vi "Heating second step (SILAR).vi"(0 "Arduino Resource In":T1={"VISA resource"="", "Board Type"=enum."Uno", "Connection Type"=enum."USB / Serial", "Bytes Per Packet (15)"=15}, 2 "Turn on_off":bool, 3 "Время всего процесса":dbl, 5 "Error In":errorcluster, 6 "Необходимая температура":dbl[](array[numeric])=[1.0, 1.0, 1.0, 1.0], 8 "Текущая температура":dbl[](array[numeric])=[1.0, 1.0, 1.0, 1.0]) -> ()   [LabVIEW 2012]
uses:
  <vilib>/LabVIEW Interface for Arduino/Type Defs/Arduino Resource.ctl
  <vilib>/LabVIEW Interface for Arduino/Type Defs/Board Type.ctl
  <vilib>/LabVIEW Interface for Arduino/LabVIEW Interface for Arduino.lvlib
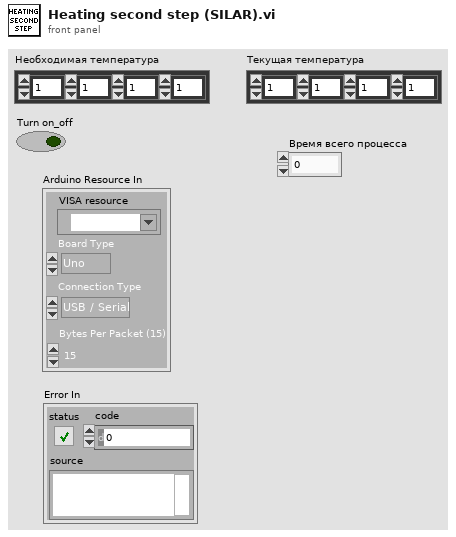
[diagram p1: front panel]
types:
  T1 = typedef "LabVIEW Interface for Arduino.lvlib/Arduino Resource.ctl" = cluster{"VISA resource":refnum<visa-resource-name>, "Board Type":T2, "Connection Type":enum8{"USB / Serial"}, "Bytes Per Packet (15)":u8}
  T2 = typedef "LabVIEW Interface for Arduino.lvlib/Board Type.ctl" = enum16{"Uno", "Dimuelanove w/Atmega 328", "Mega 2560"}
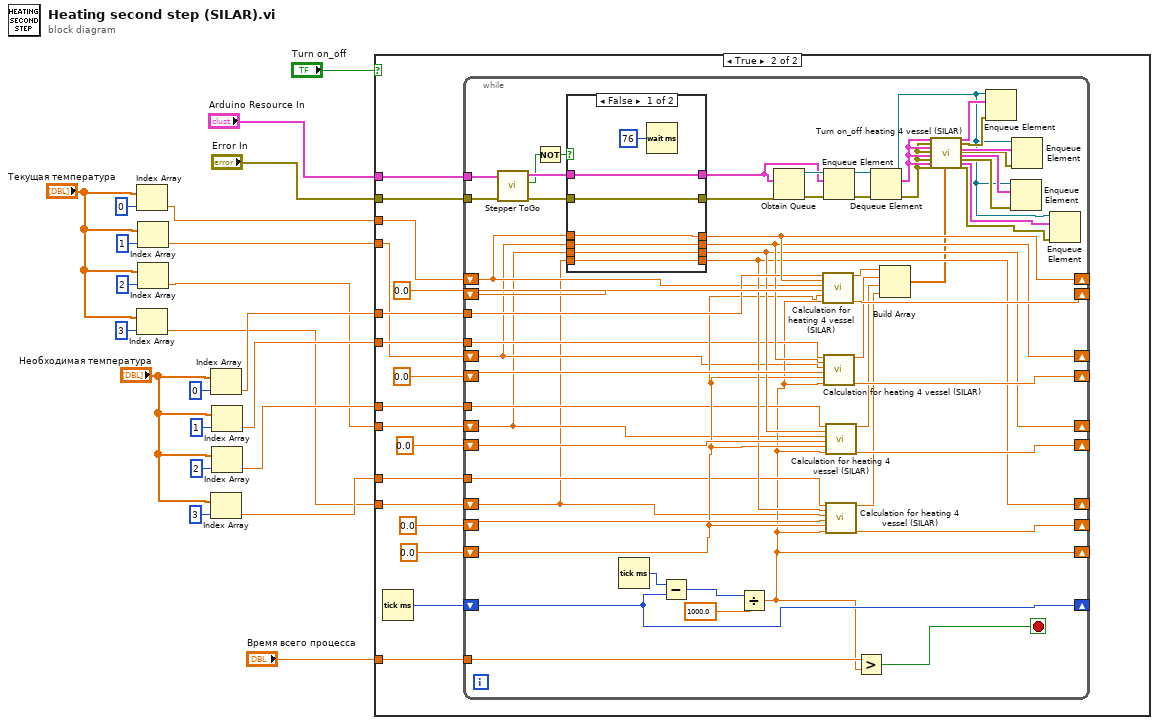
[diagram p0: block diagram]
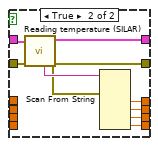
[diagram p3: hidden frame]
diagram:
  n1 = Index Array(array="Текущая температура", index=0) -> (element=w5:dbl)
  n2 = Index Array(array="Текущая температура", index=3) -> (element=w2:dbl)
  n3 = Index Array(array="Текущая температура", index=1) -> (element=w4:dbl)
  n4 = Index Array(array="Текущая температура", index=2) -> (element=w3:dbl)
  n5 = Index Array(array="Необходимая температура", index=0) -> (element=w17:dbl)
  n6 = Index Array(array="Необходимая температура", index=3) -> (element=w14:dbl)
  n7 = Index Array(array="Необходимая температура", index=1) -> (element=w16:dbl)
  n8 = Index Array(array="Необходимая температура", index=2) -> (element=w15:dbl)
  n9 = case shown="True" "Turn on_off" {
    tunnel: "Arduino Resource In" -> [_ w39]
    tunnel: "Error In" -> [_ w38]
    tunnel: w17 -> [_ w36]
    tunnel: w16 -> [_ w30]
    tunnel: w15 -> [_ w29]
    tunnel: w14 -> [_ w28]
    tunnel: w5 -> [_ w27]
    tunnel: w4 -> [_ w26]
    tunnel: w3 -> [_ w25]
    tunnel: w2 -> [_ w24]
    tunnel: "Время всего процесса" -> [_ w23]
    frame False {
    }
    frame True {
      n10 = Tick Count (ms)() -> (millisecond timer value=w35:u32)
      n11 = while {
        tunnel: w39 -> [w55]
        tunnel: w38 -> [w56]
        shift-right: [w81] -> _
        shift-left: w27 -> [w47]
        shift-right: [w83] -> _
        shift-left: 0.0 ("Ts - суммарная температура") -> [w82]
        tunnel: w36 -> [w80]
        shift-right: [w73] -> _
        shift-left: w26 -> [w46]
        shift-right: [w77] -> _
        shift-left: 0.0 -> [w76]
        shift-right: [w72] -> _
        shift-left: w25 -> [w45]
        shift-right: [w78] -> _
        shift-left: 0.0 -> [w75]
        shift-right: [w71] -> _
        shift-left: w24 -> [w44]
        shift-right: [w79] -> _
        shift-left: 0.0 -> [w74]
        shift-right: [w67] -> _
        shift-left: w35 -> [w67]
        shift-right: [w49] -> _
        shift-left: 0.0 -> [w66]
        tunnel: w30 -> [w65]
        tunnel: w29 -> [w64]
        tunnel: w28 -> [w63]
        tunnel: w23 -> [w50]
        stop <- w48 stop-if-true
        n12 = call <vilib>:"Stepper ToGo.vi"("error in"=w56, "Arduino Resource"=w55) -> ("error out"=w53:errorcluster, "Steps Remaining?"=w51:bool, "Arduino Resource Out"=w54:T1)  [unwired: 6 in, 1 out]
        n13 = Not(x=w51) -> (.not. x?=w52:bool)
        n14 = case shown="False" w52 {
          tunnel: [w101 w111] -> w94
          tunnel: [w99 w110] -> w81
          tunnel: [w98 w109] -> w73
          tunnel: [w97 w108] -> w72
          tunnel: [w96 w107] -> w71
          tunnel: [w100 w105] -> w57
          tunnel: w54 -> [w101 w104]
          tunnel: w53 -> [w100 w103]
          tunnel: w47 -> [w99 _]
          tunnel: w46 -> [w98 _]
          tunnel: w45 -> [w97 _]
          tunnel: w44 -> [w96 _]
          frame False {
            n15 = Wait (ms)(milliseconds to wait=u32 76) -> ()  [unwired: 1 out]
          }
          frame True {
            n16 = call "Reading temperature (SILAR).vi"("error in"=w103, "Arduino Resource in"=w104) -> ("error out"=w105:errorcluster, "Arduino Resource"=w111:T1, "read buffer"=w106:string)  [unwired: 7 in]
            n17 = Scan From String(input string=w106, error in=w105) -> (output 1=w110:dbl, output 2=w109:dbl, output 3=w108:dbl, output 4=w107:dbl)  [unwired: 6 in, 3 out]
          }
        }
        n18 = Tick Count (ms)() -> (millisecond timer value=w70:u32)
        n19 = Subtract(x=w70, y=w67) -> (x-y=w68:u32)
        n20 = Divide(x=w68, y=1000.0) -> (x/y=w49:dbl)
        n21 = Obtain Queue(element data type=w94, error in (no error)=w57) -> (queue out=w95:refnum<queue>, error out=w40:errorcluster)  [unwired: 3 in, 1 out]
        n22 = call "Calculation for heating 4 vessel (SILAR).vi"("Tz - заданная температура"=w80, "Tt - текущая температура"=w81, "Ttp - текущая (прошлая) температура"=w47, "Tsp - суммарная (прошлая) температура"=w82, "tp - время прошлое"=w66, "tn - время настоящее"=w49) -> ("t1 - время во включенном состоянии"=w62:dbl, "Ts - суммарная температура"=w83:dbl)  [unwired: 12 in]
        n23 = Enqueue Element(queue=w95, element=w94, error in (no error)=w40) -> (queue out=w93:refnum<queue>, error out=w92:errorcluster)  [unwired: 1 in, 1 out]
        n24 = call "Calculation for heating 4 vessel (SILAR).vi"("Tz - заданная температура"=w65, "Tt - текущая температура"=w73, "Ttp - текущая (прошлая) температура"=w46, "Tsp - суммарная (прошлая) температура"=w76, "tp - время прошлое"=w66, "tn - время настоящее"=w49) -> ("t1 - время во включенном состоянии"=w60:dbl, "Ts - суммарная температура"=w77:dbl)  [unwired: 12 in]
        n25 = call "Calculation for heating 4 vessel (SILAR).vi"("Tz - заданная температура"=w64, "Tt - текущая температура"=w72, "Ttp - текущая (прошлая) температура"=w45, "Tsp - суммарная (прошлая) температура"=w75, "tp - время прошлое"=w66, "tn - время настоящее"=w49) -> ("t1 - время во включенном состоянии"=w59:dbl, "Ts - суммарная температура"=w78:dbl)  [unwired: 12 in]
        n26 = call "Calculation for heating 4 vessel (SILAR).vi"("Tz - заданная температура"=w63, "Tt - текущая температура"=w71, "Ttp - текущая (прошлая) температура"=w44, "Tsp - суммарная (прошлая) температура"=w74, "tp - время прошлое"=w66, "tn - время настоящее"=w49) -> ("t1 - время во включенном состоянии"=w58:dbl, "Ts - суммарная температура"=w79:dbl)  [unwired: 12 in]
        n27 = Greater?(x=w50, y=w49) -> (0:w48:bool)
        n28 = Dequeue Element(queue=w93, error in (no error)=w92) -> (queue out=w41:refnum<queue>, element=w91:T1, error out=w90:errorcluster)  [unwired: 1 in, 1 out]
        n29 = Build Array(w62, w60, w59, w58) -> (w61:dbl[])
        n30 = call "Turn on_off heating 4 vessel (SILAR).vi"("Arduino Resource in 1"=w91, "Error in 1"=w90, "Arduino Resource in 2"=w91, "Error in 2"=w90, "Arduino Resource in 3"=w91, "Error in 3"=w90, "Arduino Resource in 4"=w91, "Error in 4"=w90, "t1 - время во включенном состоянии"=w61) -> ("Arduino Resource out 1"=w89:T1, "Error out 1"=w88:errorcluster, "Arduino Resource out 2"=w87:T1, "Error out 2"=w86:errorcluster, "Arduino Resource out 3"=w85:T1, "Error out 3"=w84:errorcluster, "Arduino Resource out 4"=w42:T1, "Error out 4"=w43:errorcluster)  [unwired: 11 in]
        n31 = Enqueue Element(queue=w41, element=w89, error in (no error)=w88) -> ()  [unwired: 1 in, 3 out]
        n32 = Enqueue Element(queue=w41, element=w85, error in (no error)=w84) -> ()  [unwired: 1 in, 3 out]
        n33 = Enqueue Element(queue=w41, element=w87, error in (no error)=w86) -> ()  [unwired: 1 in, 3 out]
        n34 = Enqueue Element(queue=w41, element=w42, error in (no error)=w43) -> ()  [unwired: 1 in, 3 out]
      }
    }
  }
